vi "sv_Convert String to Value (Direction).vi"(7 "direction string":string) -> (8 "direction value":T1 items=["-Z Rotation"=-6, "-Y Rotation"=-5, "-X Rotation"=-4, "-Z Translation"=-3, "-Y Translation"=-2, "-X Translation"=-1, "Scalar"=0, "+X Translation"=1, "+Y Translation"=2, "+Z Translation"=3, "+X Rotation"=4, "+Y Rotation"=5, "+Z Rotation"=6])   [LabVIEW 2017, in "SoundVib_UFF58.lvlib"]
uses:
  <vilib>/addons/Sound and Vibration/svt_UFF58/SoundVib_UFF58.lvlib
  <vilib>/addons/Sound and Vibration/svt_UFF58/subVIs/sv_UFF58 Response Direction.ctl
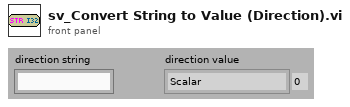
[diagram p1: front panel]
types:
  T1 = typedef "SoundVib_UFF58.lvlib/sv_UFF58 Response Direction.ctl" = i32
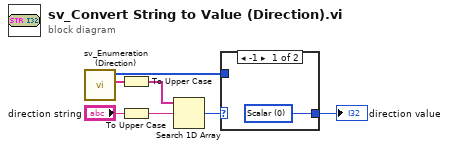
[diagram p0: block diagram]
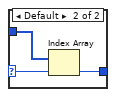
[diagram p2: hidden frame]
diagram:
  n1 = call <vilib>:"sv_Enumeration (Direction).vi"() -> ("direction strings"=w2:string[], "direction values"=w1:T1[])  [unwired: 10 in]
  n2 = To Upper Case(1:w2) -> (0:w5:string[])
  n3 = To Upper Case(1:"direction string") -> (0:w4:string)
  n4 = Search 1D Array(1D array=w5, element=w4) -> (index of element=w3:i32)  [unwired: 1 in]
  n5 = case shown="-1" w3 {
    selector: w3 -> [_ w10]
    tunnel: [w8 w9] -> w7
    tunnel: w1 -> [_ w11]
    frame -1 {
      w8 = T1 0 items=["-Z Rotation"=-6, "-Y Rotation"=-5, "-X Rotation"=-4, "-Z Translation"=-3, "-Y Translation"=-2, "-X Translation"=-1, "Scalar"=0, "+X Translation"=1, "+Y Translation"=2, "+Z Translation"=3, "+X Rotation"=4, "+Y Rotation"=5, "+Z Rotation"=6] ("ResponseDirection")
    }
    frame Default {
      n6 = Index Array(array=w11, index=w10) -> (element=w9:T1)
    }
  }
  "direction value" <- w7
